vi "main.vi"() -> ()   [LabVIEW 2020]
uses:
  <vilib>/DAQmx/read.llb/DAQmx Read (Analog 1D DBL NChan 1Samp).vi
  <vilib>/DAQmx/create/channels.llb/DAQmx Create Channel (AI-Current-Basic).vi
  <vilib>/Utility/file.llb/Write Delimited Spreadsheet (string).vi
  sub_vi/Timing.llb/getRelativeTime(Host).vi
  <vilib>/DAQmx/miscellaneous.llb/DAQmx Fill In Error Info.vi
  <vilib>/Utility/file.llb/Write Delimited Spreadsheet (DBL).vi
  sub_vi/PlotGraph.llb/Plot_Y_Graph(RelativeTime-Scope).vi
  sub_vi/PlotGraph.llb/GraphPlot.lvlib
  sub_vi/Timing.llb/Timing.lvlib
  <resource>/objmgr/daqmx.rc
panel:
  out "f2":dbl format="%.1f"
  out "f1":dbl format="%.1f"
  out "p3":dbl format="%.1f"
  out "p2":dbl format="%.1f"
  out "p1":dbl format="%.1f"
  out "flow_rate":cluster{dbl[], dbl[]}[](graph)
  out "pressure":cluster{dbl[], dbl[]}[](graph)
  in  "stop":bool
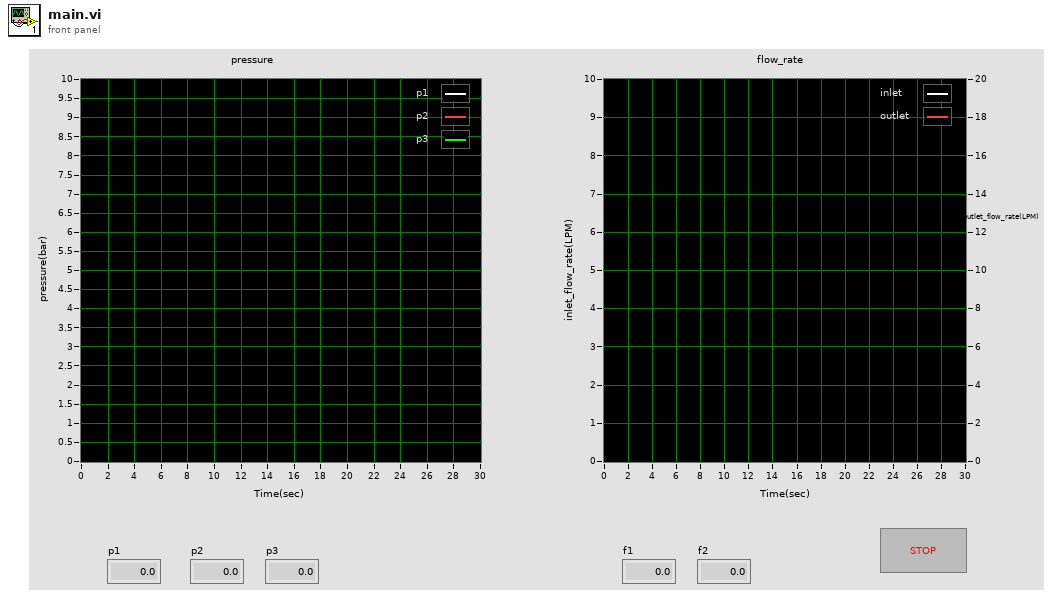
[diagram p1: front panel]
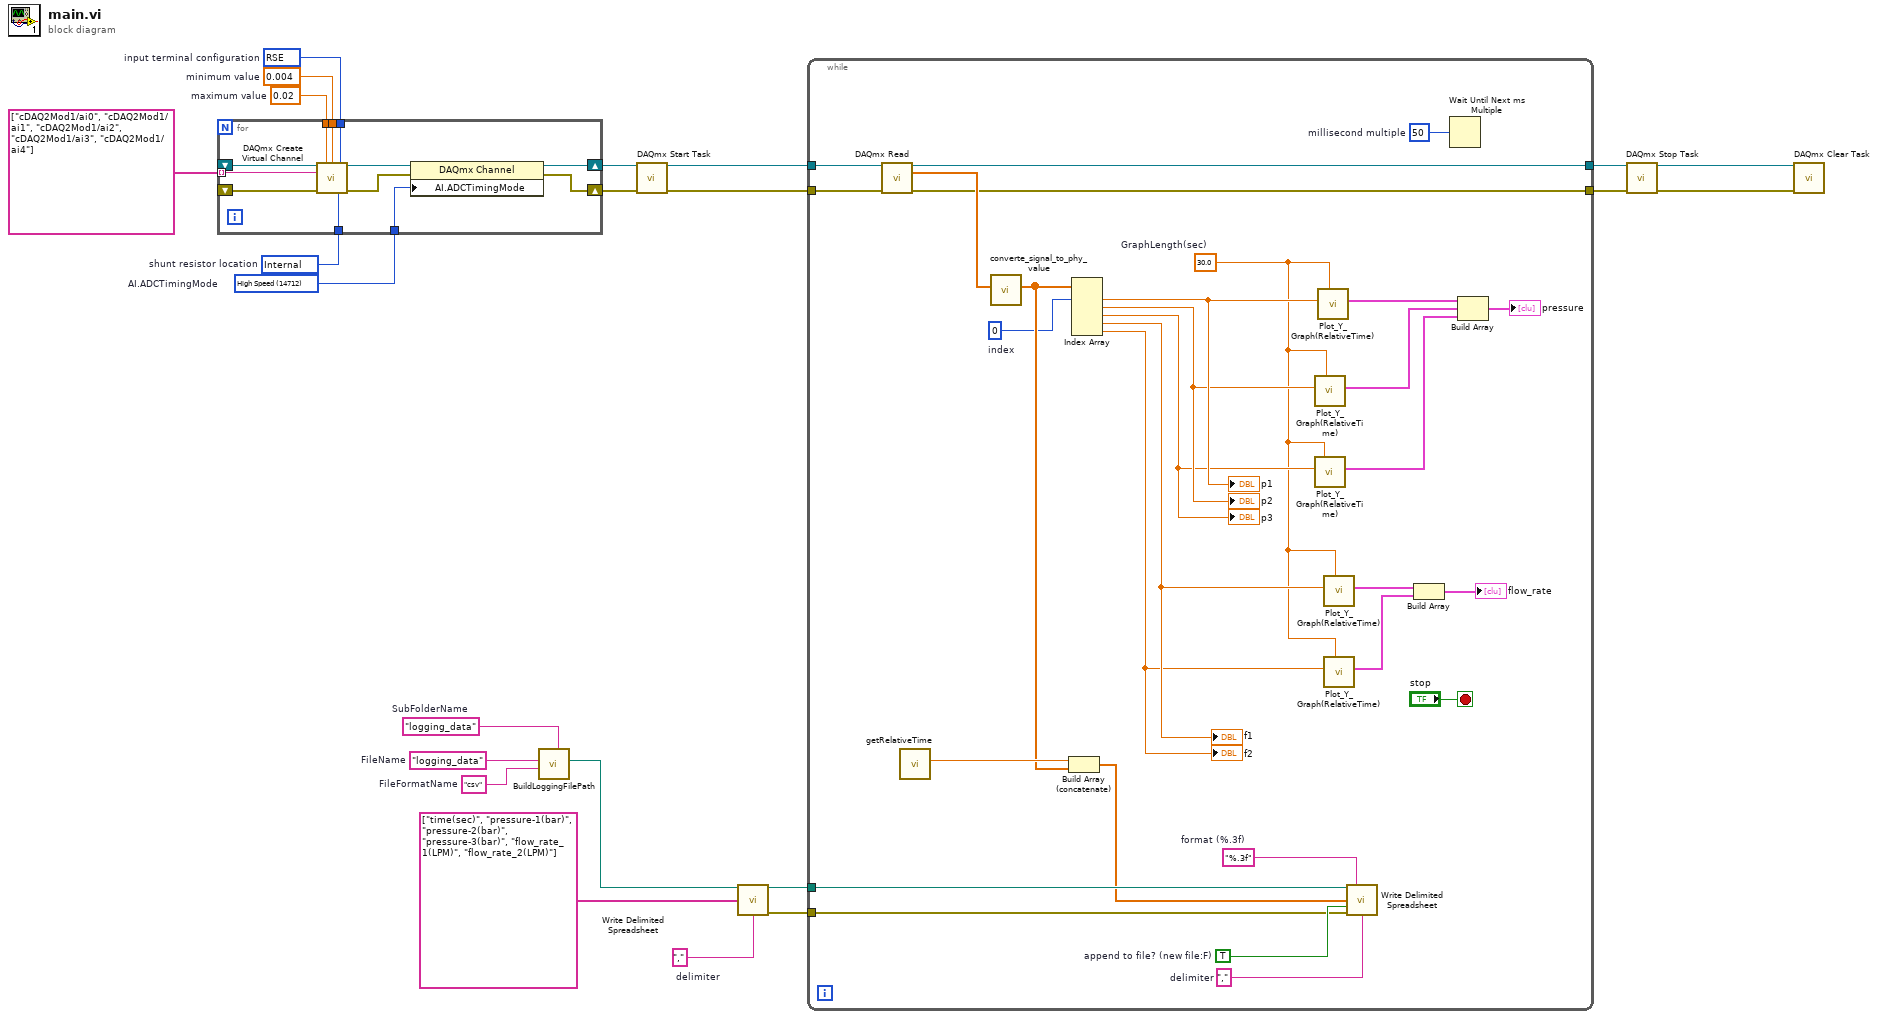
[diagram p0: block diagram]
diagram:
  w1 = "logging_data"  # SubFolderName
  w2 = "csv"  # FileFormatName
  w3 = "logging_data"  # FileName
  w11 = 14712 items=["Automatic"=16097, "High Resolution"=10195, "High Speed"=14712, "Best 50 Hz Rejection"=14713, "Best 60 Hz Rejection"=14714, "Custom"=10137]  # AI.ADCTimingMode
  w12 = 10083 items=["default"=-1, "RSE"=10083, "NRSE"=10078, "Differential"=10106, "Pseudodifferential"=12529]  # input terminal configuration
  w13 = 10200 items=["default"=-1, "Internal"=10200, "External"=10167]  # shunt resistor location
  w15 = 0.004  # minimum value
  w16 = 0.02  # maximum value
  w17 = ","  # delimiter
  n1 = for {
    tunnel: w16 -> [w34]
    tunnel: w15 -> [w33]
    tunnel: tag[] ["cDAQ2Mod1/ai0", "cDAQ2Mod1/ai1", "cDAQ2Mod1/ai2", "cDAQ2Mod1/ai3", "cDAQ2Mod1/ai4"] -> [w32] mode=indexing
    shift-right: [w24] -> w10
    shift-left: _ -> [w31]
    tunnel: w13 -> [w30]
    tunnel: w12 -> [w29]
    shift-right: [w23] -> w9
    shift-left: _ -> [w28]
    tunnel: w11 -> [w26]
    n2 = call-poly <vilib>:"DAQmx Create Virtual Channel.vi"("task in"=w31, "maximum value"=w34, "minimum value"=w33, "input terminal configuration"=w29, "physical channels"=w32, "error in"=w28, "shunt resistor location"=w30) -> ("task out"=w27:refnum<k21>, "error out"=w25:errorcluster)  [unwired: 7 in]
    n3 = property class="DAQmx Channel"(reference=w27, error in=w25, "AI.ADCTimingMode"=w26) -> (reference out=w24:refnum<k21>, error out=w23:errorcluster)
  }
  n4 = call "BuildLoggingFilePath.vi"("SubFolderName"=w1, "FileFormatName"=w2, "FileName"=w3) -> ("appended path"=w4:path)  [unwired: 8 in]
  n5 = call <vilib>:"DAQmx Start Task.vi"("task/channels in"=w10, "error in"=w9) -> ("task out"=w22:refnum<k21>, "error out"=w21:errorcluster)  [unwired: 12 in]
  n6 = call-poly <vilib>:"Write Delimited Spreadsheet.vi"("file path (dialog if empty)"=w4, "1D data"=string[] ["time(sec)", "pressure-1(bar)", "pressure-2(bar)", "pressure-3(bar)", "flow_rate_1(LPM)", "flow_rate_2(LPM)"], "delimiter (\\t)"=w17) -> ("new file path (Not A Path if cancelled)"=w20:path, "error out"=w19:errorcluster)  [unwired: 11 in]
  n7 = while {
    tunnel: w22 -> [w63]
    tunnel: w21 -> [w62]
    tunnel: w20 -> [w44]
    tunnel: w19 -> [w43]
    tunnel: [w36] -> w8
    tunnel: [w35] -> w7
    stop <- "stop" stop-if-true
    w37 = 0  # index
    w40 = 30.0  # GraphLength(sec)
    w45 = "%.3f"  # format (%.3f)
    w46 = TRUE  # append to file? (new file:F)
    w47 = ","  # delimiter
    w60 = u32 50  # millisecond multiple
    n8 = call-poly <vilib>:"DAQmx Read.vi"("task/channels in"=w63, "error in"=w62) -> ("task out"=w36:refnum<k21>, "data"=w39:dbl[], "error out"=w35:errorcluster)  [unwired: 11 in]
    n9 = call-poly "getRelativeTime.vi"() -> ("getRelativeTime(sec)"=w41:dbl)  [unwired: 11 in]
    n10 = call "converte_signal_to_phy_value.vi"("data in"=w39) -> ("data out"=w38:dbl[])  [unwired: 10 in]
    n11 = Build Array (concatenate)(w41, w38) -> (w42:dbl[])
    n12 = Index Array "Index Array"(array=w38, index #1=w37) -> (element #1=w52:dbl, element #2=w51:dbl, element #3=w50:dbl, element #4=w49:dbl, element #5=w48:dbl)  [unwired: 4 in]
    "p1" <- w52
    "p2" <- w51
    "p3" <- w50
    "f1" <- w49
    "f2" <- w48
    n13 = call-poly "Plot_Y_Graph(RelativeTime).vi"("GraphLength(sec)"=w40, "DataInput(Y-Value)"=w51) -> ("XYGraph"=w58:cluster{dbl[], dbl[]})  [unwired: 9 in]
    n14 = call-poly "Plot_Y_Graph(RelativeTime).vi"("GraphLength(sec)"=w40, "DataInput(Y-Value)"=w50) -> ("XYGraph"=w57:cluster{dbl[], dbl[]})  [unwired: 9 in]
    n15 = call-poly "Plot_Y_Graph(RelativeTime).vi"("GraphLength(sec)"=w40, "DataInput(Y-Value)"=w52) -> ("XYGraph"=w59:cluster{dbl[], dbl[]})  [unwired: 9 in]
    n16 = call-poly "Plot_Y_Graph(RelativeTime).vi"("GraphLength(sec)"=w40, "DataInput(Y-Value)"=w49) -> ("XYGraph"=w56:cluster{dbl[], dbl[]})  [unwired: 9 in]
    n17 = call-poly "Plot_Y_Graph(RelativeTime).vi"("GraphLength(sec)"=w40, "DataInput(Y-Value)"=w48) -> ("XYGraph"=w55:cluster{dbl[], dbl[]})  [unwired: 9 in]
    n18 = call-poly <vilib>:"Write Delimited Spreadsheet.vi"("file path (dialog if empty)"=w44, "format (%.3f)"=w45, "1D data"=w42, "append to file? (new file:F)"=w46, "error in (no error)"=w43, "delimiter (\\t)"=w47) -> ()  [unwired: 8 in, 2 out]
    n19 = Build Array(w56, w55) -> (→"flow_rate":cluster{dbl[], dbl[]}[])
    n20 = Wait Until Next ms Multiple(millisecond multiple=w60) -> ()  [unwired: 1 out]
    n21 = Build Array(w59, w58, w57) -> (→"pressure":cluster{dbl[], dbl[]}[])
  }
  n22 = call <vilib>:"DAQmx Stop Task.vi"("task/channels in"=w8, "error in"=w7) -> ("task out"=w6:refnum<k21>, "error out"=w5:errorcluster)  [unwired: 12 in]
  n23 = call <vilib>:"DAQmx Clear Task.vi"("task in"=w6, "error in"=w5) -> ()  [unwired: 13 in, 1 out]
